vi "Y_Scale_Change.vi"(10 "Ratio":dbl=2.0, 11 "GraphRef":refnum<vi>) -> ()   [LabVIEW 2012]
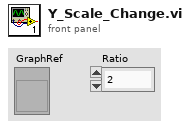
[diagram p1: front panel]
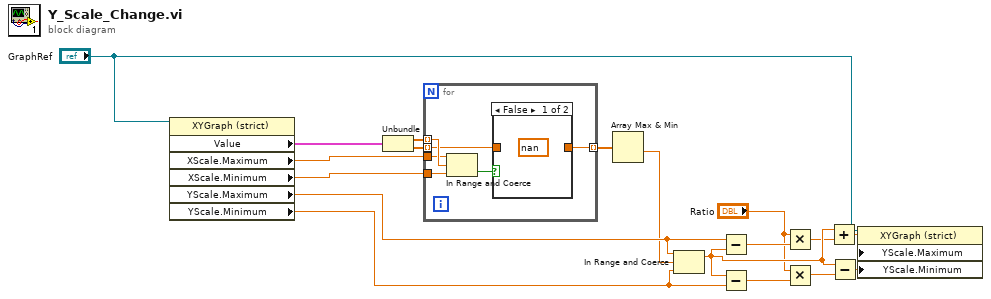
[diagram p0: block diagram]
diagram:
  n1 = property on="Property Node" class="XYGraph (strict)"(reference="GraphRef") -> ("Value"=w2:cluster{dbl[], dbl[]}, "XScale.Maximum"=w8:dbl, "XScale.Minimum"=w9:dbl, "YScale.Maximum"=w17:dbl, "YScale.Minimum"=w18:dbl)  [unwired: 1 in, 2 out]
  n2 = Unbundle(w2) -> (w6:dbl[], w7:dbl[])
  n3 = for {
    tunnel: w7 -> [w20] mode=indexing
    tunnel: w6 -> [w24] mode=indexing
    tunnel: w9 -> [w23]
    tunnel: w8 -> [w22]
    tunnel: [w19] -> w10 mode=indexing
    n4 = In Range and Coerce(upper limit=w22, x=w24, lower limit=w23) -> (In Range?=w21:bool)  [unwired: 1 out]
    n5 = case shown="False" w21 {
      tunnel: w20 -> [_ w25]
      tunnel: [_ w25] -> w19
      frame False {
        (unwired) nan
      }
      frame True {
      }
    }
  }
  n6 = Array Max & Min(array=w10) -> (min value=w16:dbl)  [unwired: 3 out]
  n7 = In Range and Coerce(upper limit=w17, x=w16, lower limit=w18) -> (coerced(x)=w15:dbl)  [unwired: 1 out]
  n8 = Subtract(x=w17, y=w15) -> (x-y=w11:dbl)
  n9 = Subtract(x=w15, y=w18) -> (x-y=w12:dbl)
  n10 = Multiply(x="Ratio", y=w11) -> (x*y=w4:dbl)
  n11 = Multiply(x="Ratio", y=w12) -> (x*y=w13:dbl)
  n12 = Add(x=w15, y=w4) -> (x+y=w5:dbl)
  n13 = Subtract(x=w15, y=w13) -> (x-y=w14:dbl)
  n14 = property on="Property Node" class="XYGraph (strict)"(reference="GraphRef", "YScale.Maximum"=w5, "YScale.Minimum"=w14) -> ()  [unwired: 1 in, 2 out]
